vi "Test_Call Measure.vi"() -> ()   [LabVIEW 2020, in "Measurement_lv_client.lvlib" / "Measurement_lv_client.lvclass"]
uses:
  Measurement_lv_client.lvclass
  RPC Messages/Measurement_v1_MeasureResponse/Measurement_v1_MeasureResponse_Data.ctl
  RPC Messages/google_protobuf_Any/google_protobuf_Any_Data.ctl
  RPC Messages/Measurement_v1_ErrorInformation/Measurement_v1_ErrorInformation_Data.ctl
  <vilib>/gRPC/LabVIEW gRPC Library/Server API/typeDefs/Message Element Type.ctl
  RPC Messages/Measurement_v1_MeasureRequest/Measurement_v1_MeasureRequest_Data.ctl
  ec24d7d7-b60a-4df4-be9f-2ccefa676409.vi
  8f422d74-d524-4bdb-aa7e-fa018c2bde97.vi
  b4d3359e-339e-42f3-8c06-4b88e853c1db.vi
  <vilib>/gRPC/LabVIEW gRPC Library/Server API/Server/Get Server DLL Path.vi
  <vilib>/gRPC/LabVIEW gRPC Library/gprc-lvsupport-release.lvlib
panel:
  out "Buffer":u8[](array[numeric])
  out "Response Data":T1
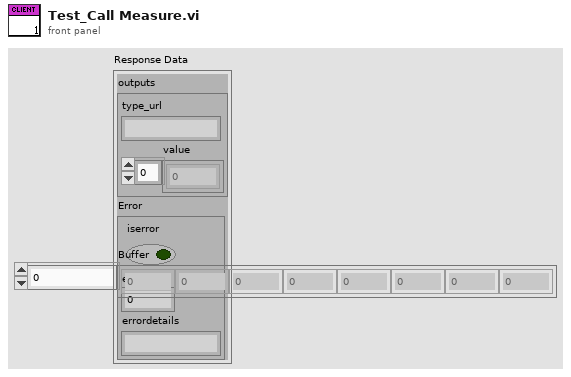
[diagram p1: front panel]
types:
  T1 = typedef "Measurement_lv_client.lvlib/Measurement_lv_client.lvclass/Measurement_v1_MeasureResponse_Data.ctl" = cluster{"outputs":T2, "Error":T3}
  T2 = typedef "Measurement_lv_client.lvlib/Measurement_lv_client.lvclass/google_protobuf_Any_Data.ctl" = cluster{"type_url":string, "value":u8[]}
  T3 = typedef "Measurement_lv_client.lvlib/Measurement_lv_client.lvclass/Measurement_v1_ErrorInformation_Data.ctl" = cluster{"iserror":bool, "errorcode":i32, "errordetails":string}
  T4 = typedef "gprc-lvsupport-release.lvlib/Message Element Type.ctl" = enum32{"Int32Value", "FloatValue", "DoubleValue", "BoolValue", "StringValue", "MessageValue", "Int64Value", "UInt32Value", "UInt64Value", "EnumValue", "Bytes", "Fixed64", "Fixed32", "SFixed64", "SFixed32", "SInt64", "SInt32"}
  T5 = typedef "gprc-lvsupport-release.lvlib/grpcId.ctl" = u64
  T6 = typedef "Measurement_lv_client.lvlib/Measurement_lv_client.lvclass/Measurement_v1_MeasureRequest_Data.ctl" = cluster{"configuration_arguments":T2}
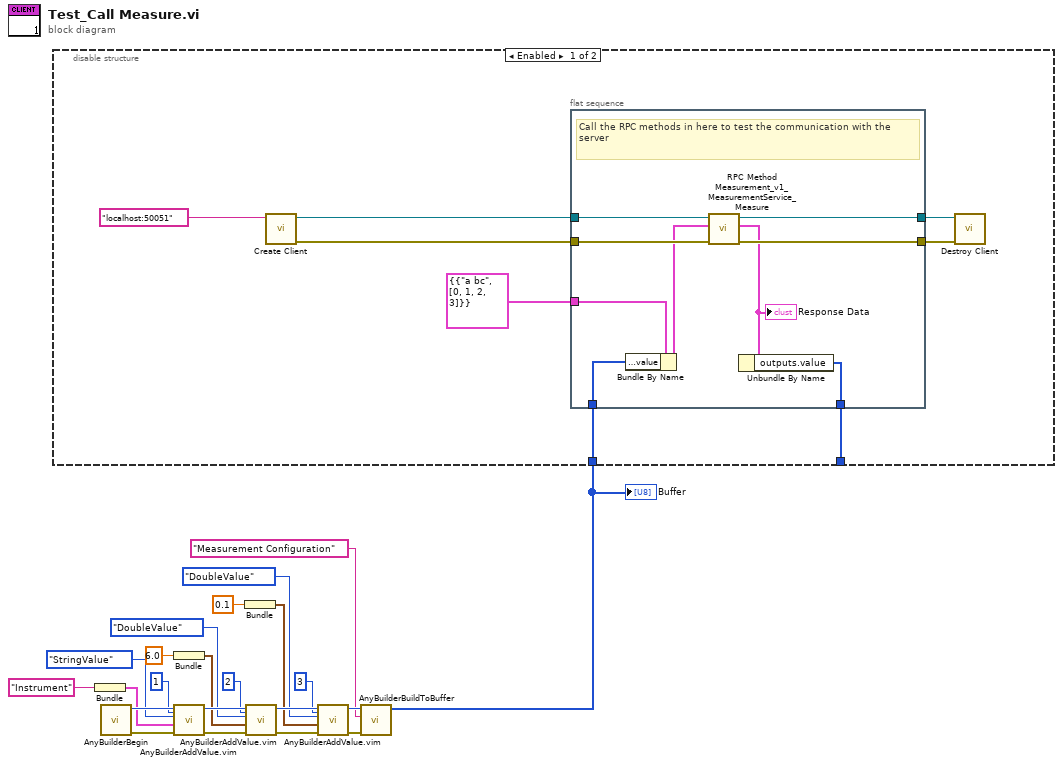
[diagram p0: block diagram]
diagram:
  n1 = Bundle("Instrument") -> (w1:cluster{string})  [unwired: 1 in]
  n2 = call <vilib>:"AnyBuilderBegin.vi"() -> ("error out"=w21:errorcluster, "Builder Ref Out"=w22:T5)  [unwired: 9 in]
  n3 = Bundle(6.0) -> (w4:cluster{dbl})  [unwired: 1 in]
  n4 = call "AnyBuilderAddValue.vim"("protobufId"=1, "error in (no error)"=w21, "Value"=w1, "MessageElementType"=Message_Element_Type."StringValue", "gRPCid in"=w22) -> ("error out"=w17:errorcluster, "gRPCid"=w18:u64)  [unwired: 5 in]
  n5 = Bundle(0.1) -> (w2:cluster{dbl})  [unwired: 1 in]
  n6 = call "AnyBuilderAddValue.vim"("protobufId"=2, "error in (no error)"=w17, "Value"=w4, "MessageElementType"=Message_Element_Type."DoubleValue", "gRPCid in"=w18) -> ("error out"=w15:errorcluster, "gRPCid"=w16:u64)  [unwired: 5 in]
  n7 = call "AnyBuilderAddValue.vim"("protobufId"=3, "error in (no error)"=w15, "Value"=w2, "MessageElementType"=Message_Element_Type."DoubleValue", "gRPCid in"=w16) -> ("error out"=w9:errorcluster, "gRPCid"=w10:u64)  [unwired: 5 in]
  n8 = call <vilib>:"AnyBuilderBuildToBuffer.vi"("error in (no error)"=w9, "Message Type"="Measurement Configuration", "Builder Ref"=w10) -> ("Buffer"=w7:u8[])  [unwired: 7 in, 1 out]
  "Buffer" <- w7
  n9 = disable-structure shown="Enabled" {
    disable-tunnel: w7 -> [w25 _]
    disable-tunnel: [w23 _] -> _
    frame Enabled {
      n10 = call "Create Client.vi"("address"="localhost:50051") -> ("error out"=w26:errorcluster, "gRPC Client out"=w28:refnum<class "Measurement_lv_client.lvclass">)  [unwired: 9 in]
      n11 = flat-sequence {
        tunnel: [w38] -> w29
        tunnel: w28 -> [w39]
        tunnel: [w36] -> w27
        tunnel: w26 -> [w37]
        tunnel: w25 -> [w33]
        tunnel: T6 {"configuration_arguments"={"type_url"="a bc", "value"=[0, 1, 2, 3]}} ("Request Data") -> [w35]
        tunnel: [w31] -> w23
        frame #0 {
          # "Call the RPC methods in here to test the communication with the server"
          n12 = Bundle By Name(cluster=w35, "configuration_arguments.value"=w33) -> (w34:T6)
          n13 = call "RPC Method Measurement_v1_MeasurementService_Measure.vi"("error in (no error)"=w37, "Request Data"=w34, "gRPC Client in"=w39) -> ("error out"=w36:errorcluster, "Response Data"=w32:T1, "gRPC Client out"=w38:refnum<class "Measurement_lv_client.lvclass">)  [unwired: 6 in]
          "Response Data" <- w32
          n14 = Unbundle By Name(w32) -> ("outputs.value"=w31:u8[])
        }
      }
      n15 = call "Destroy Client.vi"("error in (no error)"=w27, "gRPC Client in"=w29) -> ()  [unwired: 8 in, 2 out]
    }
    frame Disabled {
    }
  }
